vi "Grid_Write Status.vi"(10 "Grid_Status":cluster{"kW":dbl}, 11 "Grid in":refnum<class "Grid.lvclass">) -> (3 "Grid out":refnum<class "Grid.lvclass">)   [LabVIEW 2015, in "Grid.lvclass"]
uses:
  Grid.lvclass
  Grid.lvclass/Grid.ctl
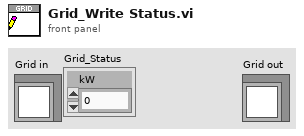
[diagram p1: front panel]
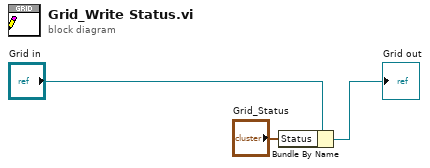
[diagram p0: block diagram]
diagram:
  n1 = Bundle By Name(cluster="Grid in", "Status"="Grid_Status") -> (→"Grid out":refnum<class "Grid.lvclass">)
